vi "Day 21.vi"() -> ()   [LabVIEW 2021]
panel:
  out "x*y":i32
  in  "Input File":enum32{"example input", "input"}(radio)
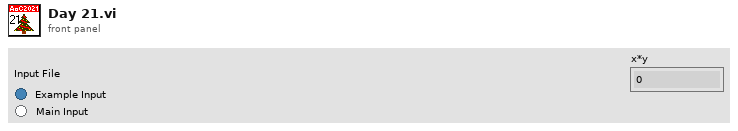
[diagram p1: front panel]
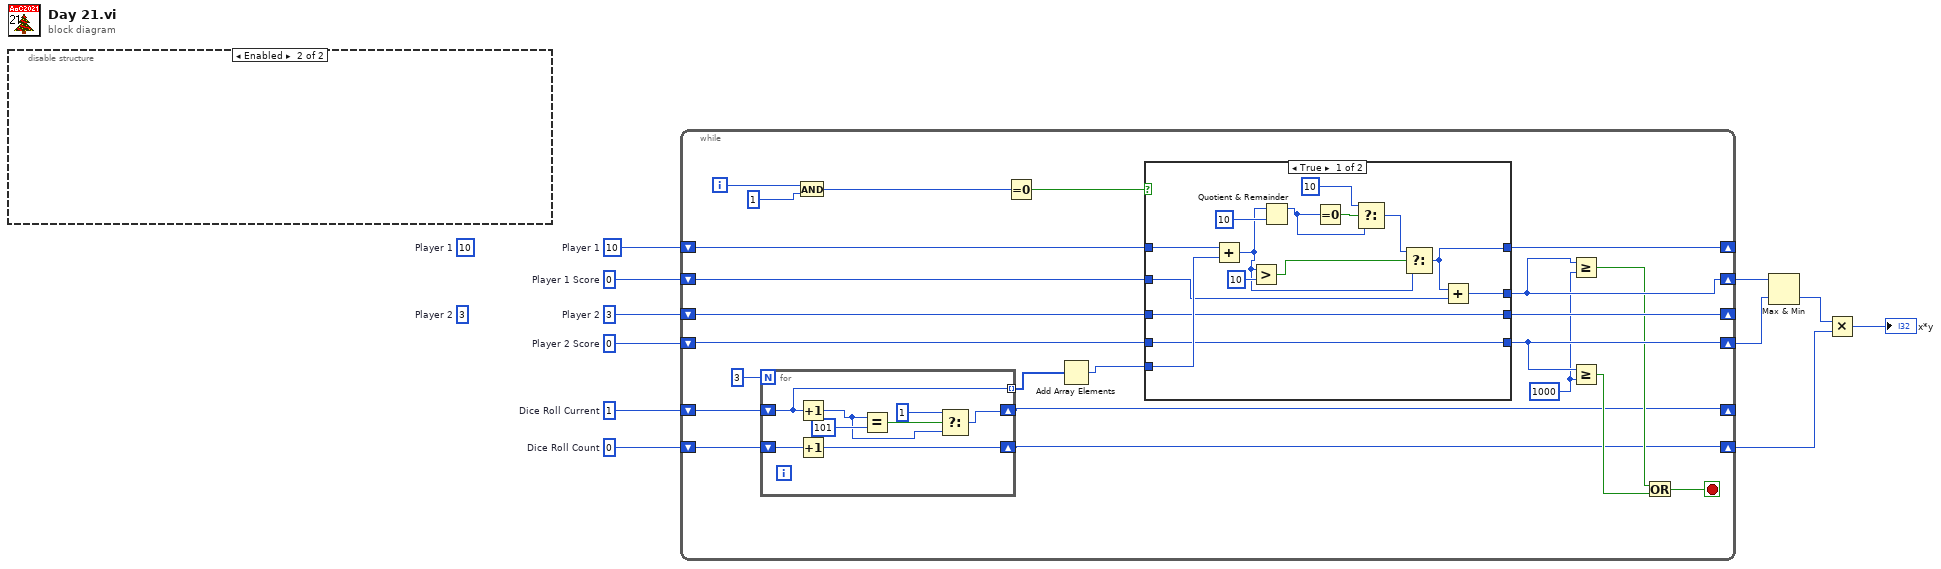
[diagram p0: block diagram]
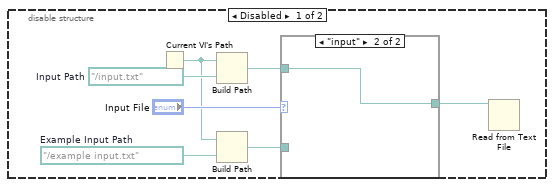
[diagram p2: hidden frame]
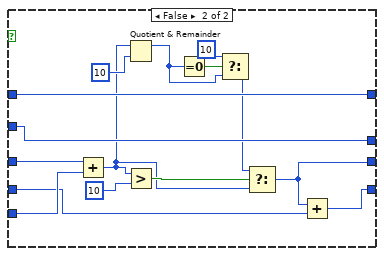
[diagram p4: hidden frame]
diagram:
  (unwired) 3  # Player 2
  (unwired) 10  # Player 1
  w6 = u64 0  # Player 2 Score
  w7 = u64 0  # Player 1 Score
  w8 = u64 1  # Dice Roll Current
  w9 = u64 0  # Dice Roll Count
  w10 = u64 3  # Player 2
  w11 = u64 10  # Player 1
  n1 = disable-structure shown="Enabled" {
    frame Disabled {
      w17 = path "../example input.txt"  # Example Input Path
      w18 = path "../input.txt"  # Input Path
      n2 = Current VI's Path() -> (path=w12:path)
      n3 = Build Path(base path=w12, name or relative path=w18) -> (appended path=w15:path)
      n4 = Build Path(base path=w12, name or relative path=w17) -> (appended path=w14:path)
      n5 = case shown="\"input\"" "Input File" {
        tunnel: w15 -> [_ w20]
        tunnel: w14 -> [w19 _]
        tunnel: [w19 w20] -> w13
        frame "example input" {
        }
        frame "input" {
        }
      }
      n6 = Read from Text File(file (use dialog)=w13) -> ()  [unwired: 3 in, 4 out]
    }
    frame Enabled {
    }
  }
  n7 = while {
    shift-right: [w36] -> _
    shift-left: w11 -> [w39]
    shift-right: [w35] -> _
    shift-left: w10 -> [w38]
    shift-right: [w25] -> w2
    shift-left: w9 -> [w26]
    shift-right: [w22] -> _
    shift-left: w8 -> [w27]
    shift-right: [w33] -> w5
    shift-left: w7 -> [w37]
    shift-right: [w32] -> w4
    shift-left: w6 -> [w34]
    i -> [w43]
    stop <- w28 stop-if-true
    w31 = u64 1000
    n8 = for {
      N: 3 -> [_]
      shift-right: [w44] -> w22
      shift-left: w27 -> [w45]
      shift-right: [w50] -> w25
      shift-left: w26 -> [w51]
      tunnel: [w45] -> w24 mode=indexing
      n9 = Increment(x=w45) -> (x+1=w47:u64)
      n10 = Increment(x=w51) -> (x+1=w50:u64)
      n11 = Equal?(x=w47, y=u64 101) -> (x = y?=w48:bool)
      n12 = Select(t=u64 1, s=w48, f=w47) -> (s? t:f=w44:u64)
    }
    n13 = And(x=w43, y=1) -> (x .and. y?=w41:i32)
    n14 = Equal To 0?(x=w41) -> (x = 0?=w40:bool)
    n15 = Add Array Elements(numeric array=w24) -> (sum=w23:u64)
    n16 = case shown="True" w40 {
      tunnel: w39 -> [w66 w75]
      tunnel: w38 -> [w62 w79]
      tunnel: w23 -> [w65 w81]
      tunnel: w37 -> [w64 w76]
      tunnel: [w63 w76] -> w33
      tunnel: [w56 w75] -> w36
      tunnel: [w62 w71] -> w35
      tunnel: [w61 w77] -> w32
      tunnel: w34 -> [w61 w78]
      frame True {
        n17 = Add(x=w66, y=w65) -> (x+y=w57:u64)
        n18 = Greater?(x=w57, y=u64 10) -> (0:w58:bool)
        n19 = Quotient & Remainder(x=w57, y=u64 10) -> (x-y*floor(x/y)=w53:u64)  [unwired: 1 out]
        n20 = Equal To 0?(x=w53) -> (x = 0?=w55:bool)
        n21 = Select(t=u64 10 ("y"), s=w55, f=w53) -> (s? t:f=w52:u64)
        n22 = Select(t=w52, s=w58, f=w57) -> (s? t:f=w56:u64)
        n23 = Add(x=w56, y=w64) -> (x+y=w63:u64)
      }
      frame False {
        n24 = Add(x=w79, y=w81) -> (x+y=w72:u64)
        n25 = Quotient & Remainder(x=w72, y=u64 10) -> (x-y*floor(x/y)=w68:u64)  [unwired: 1 out]
        n26 = Greater?(x=w72, y=u64 10) -> (0:w73:bool)
        n27 = Equal To 0?(x=w68) -> (x = 0?=w70:bool)
        n28 = Select(t=u64 10, s=w70, f=w68) -> (s? t:f=w67:u64)
        n29 = Select(t=w67, s=w73, f=w72) -> (s? t:f=w71:u64)
        n30 = Add(x=w71, y=w78) -> (x+y=w77:u64)
      }
    }
    n31 = Greater Or Equal?(x=w33, y=w31) -> (x >= y?=w30:bool)
    n32 = Greater Or Equal?(x=w32, y=w31) -> (x >= y?=w29:bool)
    n33 = Or(x=w30, y=w29) -> (x .or. y?=w28:bool)
  }
  n34 = Max & Min(x=w5, y=w4) -> (min(x,y)=w3:u64)  [unwired: 1 out]
  n35 = Multiply(x=w3, y=w2) -> (x*y=→"x*y":u64)
